vi "GetInitialPosition.vi"(8 "error in (no error)":errorcluster, 11 "reference in":refnum<class "SceneObject.lvclass">) -> (0 "error out":errorcluster, 2 "InitialPosition":T1, 3 "reference out":refnum<class "SceneObject.lvclass">)   [LabVIEW 2010, in "RenderBase.lvlib" / "SceneObject.lvclass"]
doc: "The initial position of the scene object."
uses:
  SceneObject.lvclass
  <vilib>/Utility/miscctls.llb/LV3DPointTypeDef.ctl
  SceneObject.lvclass/SceneObject.ctl
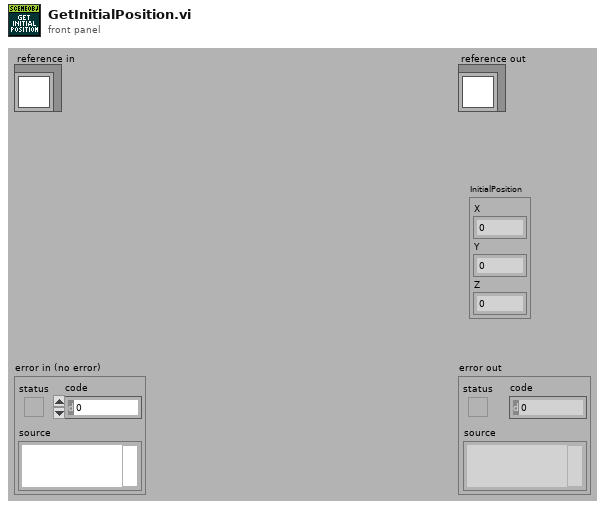
[diagram p1: front panel]
types:
  T1 = typedef "LV3DPointTypeDef.ctl" = cluster{"X":sgl, "Y":sgl, "Z":sgl}
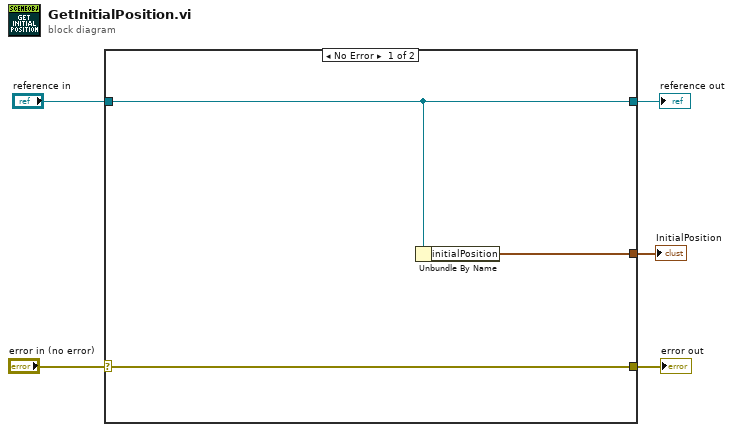
[diagram p0: block diagram]
diagram:
  n1 = case shown="No Error" "error in (no error)" {
    selector: "error in (no error)" -> [w6 w10]
    tunnel: [w6 w10] -> w4
    tunnel: [w8 w9] -> w2
    tunnel: "reference in" -> [w8 w9]
    tunnel: [w7 _] -> w1
    frame No Error {
      n2 = Unbundle By Name(w8) -> ("initialPosition"=w7:T1)
    }
    frame Error {
    }
  }
  "error out" <- w4
  "reference out" <- w2
  "InitialPosition" <- w1
